vi "Setup UI.vi"(8 "error in (no error)":errorcluster, 10 "Set UI to input? (F)":bool, 11 "Translation Stage Fine in":refnum<class "Translation Stage Fine.lvclass">) -> (0 "error out":errorcluster, 3 "Translation Stage Fine out":refnum<class "Translation Stage Fine.lvclass">)   [LabVIEW 2017, in "Translation Stage Fine.lvclass"]
doc: "Scanner::Setup is a constructor that has no parameters and faces the user. The Factory calls this VI to let the user configure this Scanner. It is dynamically dispatched in order to let the user choose the type as well as the options of the scanner."
uses:
  Translation Stage Fine.lvclass
  Global/GPIB Numbers.vi
panel:
  in  "Calibrate Zero":bool
  in  "Go to first point":bool
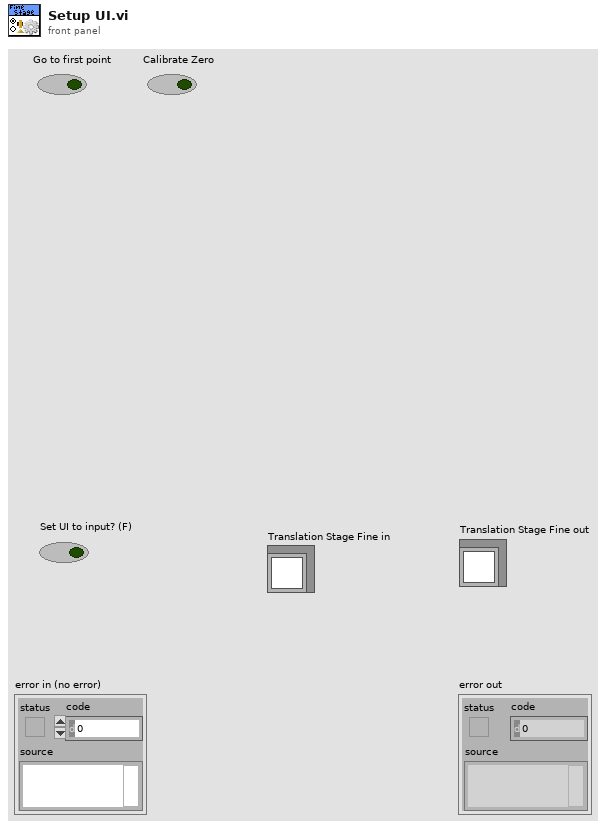
[diagram p1: front panel]
types:
  T1 = typedef "GPIB Type Def.ctl" = cluster{"Name":string, "bus":dbl, "GPIB":dbl, "GPIB as string":string, "byte":i32, "VISA Resource Name":refnum<visa-resource-name>}
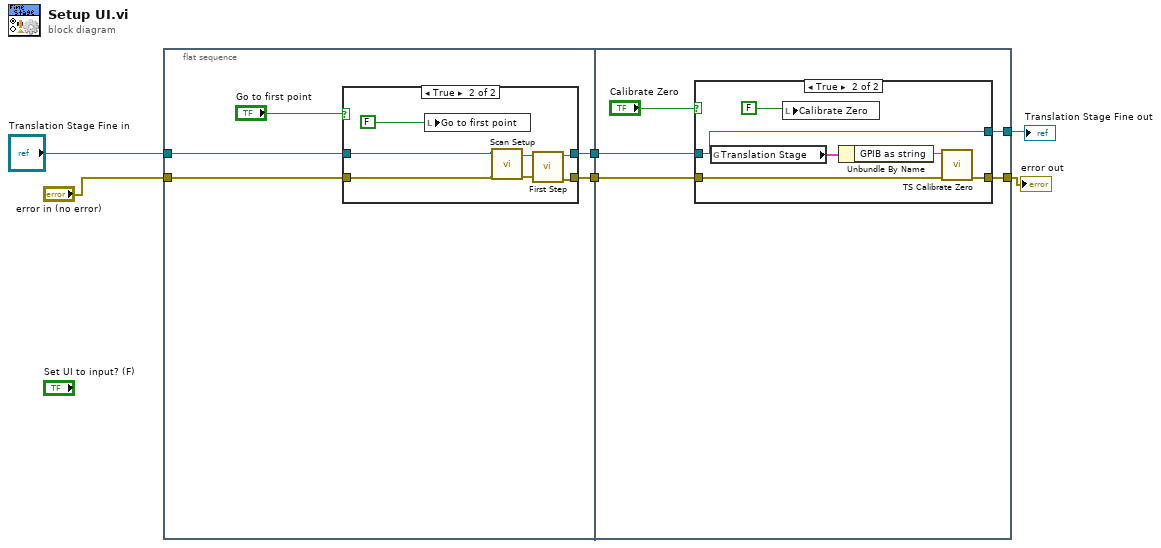
[diagram p0: block diagram]
diagram:
  n1 = flat-sequence {
    tunnel: [w11] -> w6
    tunnel: [w10] -> w5
    tunnel: "Translation Stage Fine in" -> [w8]
    tunnel: "error in (no error)" -> [w7]
    tunnel: [w24] -> w4
    tunnel: [w22] -> w2
    tunnel: w6 -> [w23]
    tunnel: w5 -> [w25]
    frame #0 {
      n2 = case shown="True" "Go to first point" {
        tunnel: [w12 w14] -> w11
        tunnel: [w13 w16] -> w10
        tunnel: w8 -> [w13 w19]
        tunnel: w7 -> [w12 w18]
        frame False {
        }
        frame True {
          n3 = local write "Go to first point"(FALSE ("Send conds for first point to PG")) -> ()
          n4 = call-dynamic "Scan Setup.vi"("error in (no error)"=w18, "Translation Stage Fine in"=w19) -> ("error out"=w15:errorcluster, "Translation Stage Fine out"=w17:refnum<class "Translation Stage Fine.lvclass">)  [unwired: 8 in]
          n5 = call-dynamic "First Step.vi"("error in (no error)"=w15, "Translation Stage Fine.lvclass in"=w17) -> ("error out"=w14:errorcluster, "Translation Stage Fine.lvclass out"=w16:refnum<class "Translation Stage Fine.lvclass">)  [unwired: 7 in, 1 out]
        }
      }
    }
    frame #1 {
      n6 = case shown="True" "Calibrate Zero" {
        tunnel: [w27 w29] -> w22
        tunnel: [w26 w30] -> w24
        tunnel: w25 -> [w26 w30]
        tunnel: w23 -> [w27 w31]
        frame False {
        }
        frame True {
          n7 = global read "GPIB Numbers.vi" "Translation Stage"() -> (w33:T1)
          n8 = local write "Calibrate Zero"(FALSE ("Send conds for first point to PG")) -> ()
          n9 = Unbundle By Name(w33) -> ("GPIB as string"=w32:string)
          n10 = call "TS Calibrate Zero.vi"("error out"=w31, "GPIB as string"=w32) -> ("error out 2"=w29:errorcluster)  [unwired: 9 out]
        }
      }
    }
  }
  "error out" <- w2
  "Translation Stage Fine out" <- w4
